vi "Periodic Tasks.vi"(8 "error in":errorcluster) -> ()   [LabVIEW 2018]
doc: "This VI runs in parallel to other tasks. It can contain as many user-defined periodic loops as you need. These can carry out PID or other sorts of timed response."
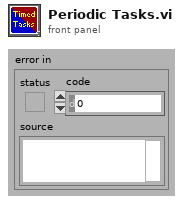
[diagram p1: front panel]
types:
  T1 = typedef "CTRE_PigeonIMU_DeviceRef.ctl" = cluster{"DeviceStatus":errorcluster, "Device Number":u8, "Type":T2, "Device ID":u32, "Handle":u64, "UsageFrame":u32, "Library Path":path}
  T2 = typedef "CTRE_PigeonIMU_ConnectionType.ctl" = u32
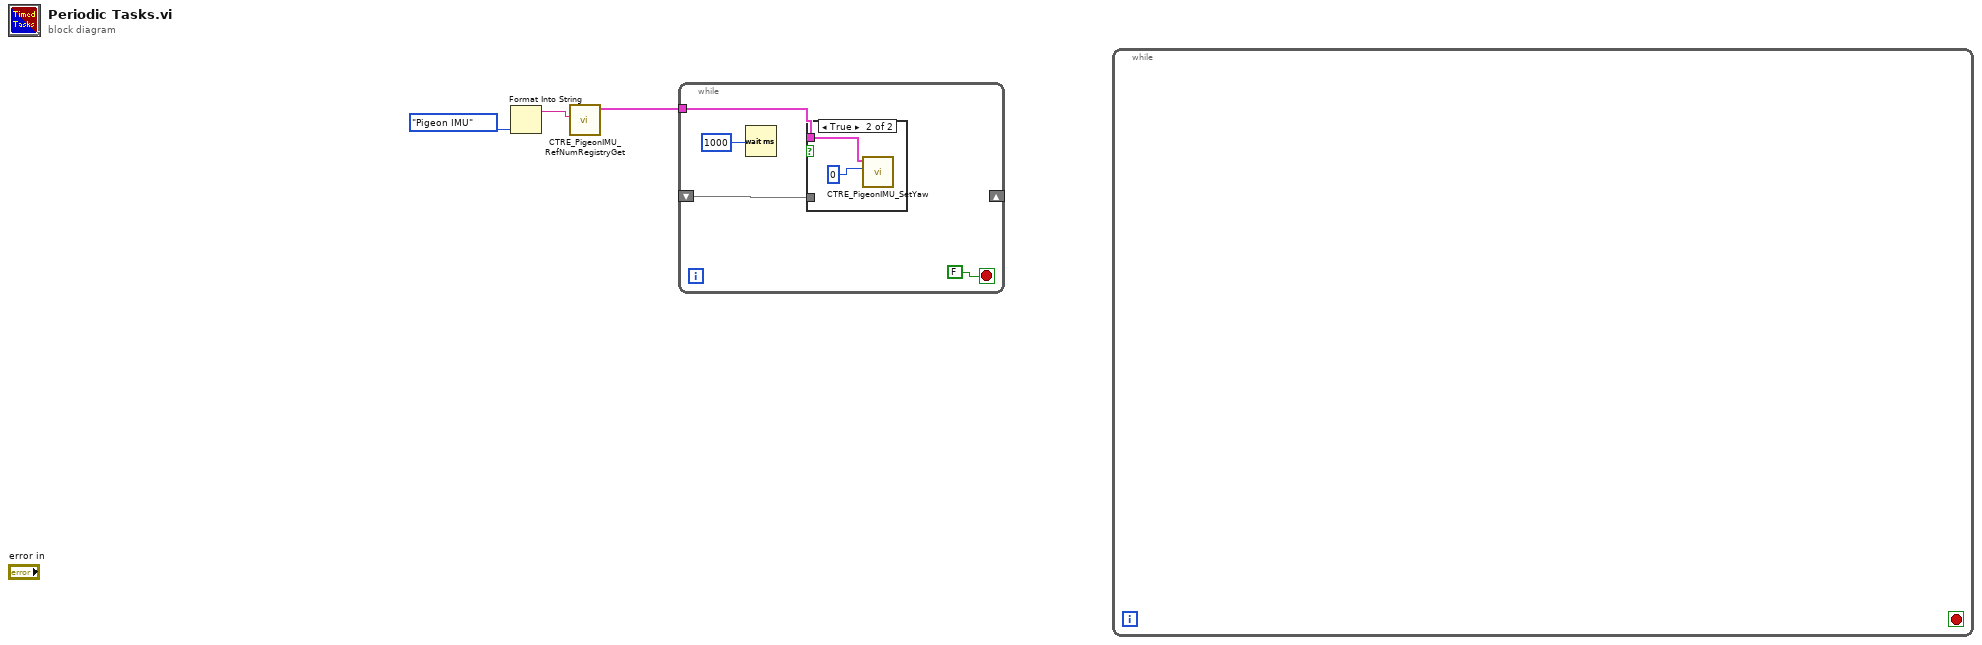
[diagram p0: block diagram]
diagram:
  n1 = Format Into String(enum16{"Pigeon IMU"}."Pigeon IMU") -> (resulting string=w2:string)  [unwired: 3 in, 1 out]
  n2 = call <vilib>:"CTRE_PigeonIMU_RefNumRegistryGet.vi"("refnum name"=w2) -> ("PigeonIMUDevRef"=w1:T1)  [unwired: 9 in, 1 out]
  n3 = while {
    tunnel: w1 -> [w5]
    shift-right: _ -> [_]
    shift-left: _ -> [w4]
    stop <- FALSE stop-if-true
    n4 = Wait (ms)(milliseconds to wait=1000) -> ()  [unwired: 1 out]
    n5 = case shown="True" {
      selector: _ -> [_ _]
      tunnel: w5 -> [_ w8]
      tunnel: w4 -> [_ _]
      frame False {
      }
      frame True {
        n6 = call <vilib>:"CTRE_PigeonIMU_SetYaw.vi"("Value"=0, "PigeonIMUDevRef"=w8) -> ()  [unwired: 8 in, 2 out]
      }
    }
  }
  n7 = while {
    stop <- _ stop-if-true
  }
